vi "data_headers_subVI.vi"(8 "Experiment Notes":string, 10 "Sample names":T1={"QCM1 sample name"="aQCM2", "QCM2 sample name"="aQCM2", "QCM3 sample name"="aQCM3", "QCM4 sample name"="aQCM4", "QCM5 sample name"="aQCM5", "QCM6 sample name"="aQCM6", "SRS sample name"="sample_SRS", "Keithley 2420 sample name"="Keithley2420", "Keithley 6430 sample name"="Keithley6430", "Keithley 2100 sample name"="Keithley6430"}) -> (2 "data headers":string[](array[string]))   [LabVIEW 2014]
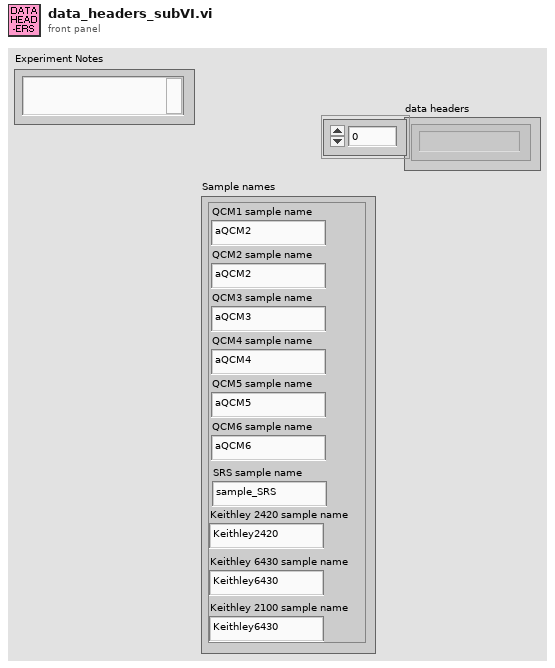
[diagram p1: front panel]
types:
  T1 = cluster{"QCM1 sample name":string, "QCM2 sample name":string, "QCM3 sample name":string, "QCM4 sample name":string, "QCM5 sample name":string, "QCM6 sample name":string, "SRS sample name":string, "Keithley 2420 sample name":string, "Keithley 6430 sample name":string, "Keithley 2100 sample name":string}
  T2 = cluster{string, string, string, string, string, string}
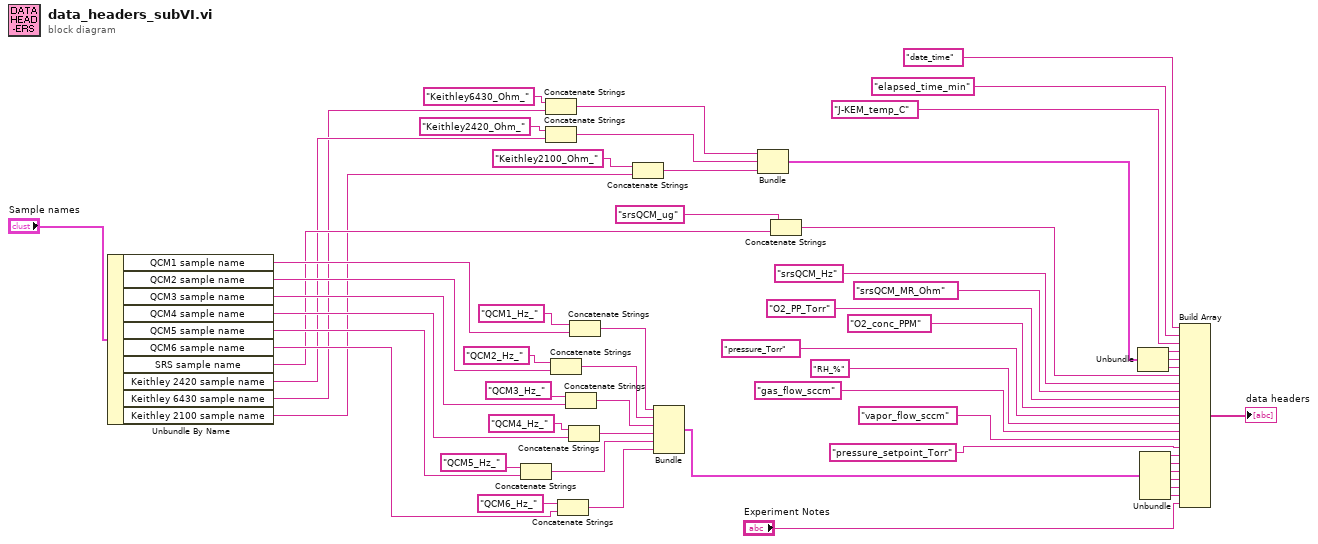
[diagram p0: block diagram]
diagram:
  n1 = Unbundle By Name("Sample names") -> ("QCM1 sample name"=w41:string, "QCM2 sample name"=w38:string, "QCM3 sample name"=w36:string, "QCM4 sample name"=w34:string, "QCM5 sample name"=w31:string, "QCM6 sample name"=w30:string, "SRS sample name"=w27:string, "Keithley 2420 sample name"=w26:string, "Keithley 6430 sample name"=w25:string, "Keithley 2100 sample name"=w23:string)
  n2 = Concatenate Strings("QCM5_Hz_" ("string"), w31) -> (w10:string)
  n3 = Concatenate Strings("Keithley6430_Ohm_", w25) -> (w21:string)
  n4 = Concatenate Strings("Keithley2420_Ohm_" ("element"), w26) -> (w20:string)
  n5 = Concatenate Strings("QCM2_Hz_" ("string"), w38) -> (w13:string)
  n6 = Concatenate Strings("QCM6_Hz_" ("string"), w30) -> (w9:string)
  n7 = Concatenate Strings("QCM3_Hz_" ("string"), w36) -> (w12:string)
  n8 = Concatenate Strings("QCM4_Hz_" ("string"), w34) -> (w11:string)
  n9 = Concatenate Strings("QCM1_Hz_" ("string"), w41) -> (w14:string)
  n10 = Concatenate Strings("Keithley2100_Ohm_" ("element"), w23) -> (w19:string)
  n11 = Bundle(w14, w13, w12, w11, w10, w9) -> (w8:T2)  [unwired: 1 in]
  n12 = Bundle(w21, w20, w19) -> (w18:cluster{string, string, string})  [unwired: 1 in]
  n13 = Concatenate Strings("srsQCM_ug", w27) -> (w28:string)
  n14 = Unbundle(w18) -> (w17:string, w16:string, w15:string)
  n15 = Unbundle(w8) -> (w2:string, w7:string, w6:string, w5:string, w4:string, w3:string)
  n16 = Build Array("date_time", "elapsed_time_min", "J-KEM_temp_C", w17, w16, w15, w28, "srsQCM_Hz", "srsQCM_MR_Ohm", "O2_PP_Torr" ("element"), "O2_conc_PPM" ("element"), "pressure_Torr" ("element"), "RH_%" ("element"), "gas_flow_sccm" ("element"), "vapor_flow_sccm" ("element"), "pressure_setpoint_Torr" ("element"), w2, w7, w6, w5, w4, w3, "Experiment Notes") -> (→"data headers":string[])
